vi "GTCP331-200ER - 1.C.(11).vi"(8 "error in (no error)":errorcluster, 11 "RT - Analysis Data in in in":T1={"Accel Sensistivity"=[0.0, 0.0, 0.0], "Cutoff Frequncies"=[{"LP Passband"=0.0, "HP Stopband"=0.0, "LP Stopband"=0.0, "HP Passband"=0.0}, {"LP Passband"=0.0, "HP Stopband"=0.0, "LP Stopband"=0.0, "HP Passband"=0.0}, {"LP Passband"=0.0, "HP Stopband"=0.0, "LP Stopband"=0.0, "HP Passband"=0.0}], "APU Setup File"={"Sensor Info"=[], "Calibration Info"=[], "CMM Table 106"=[], "CMM Table 106B "=[], "Accel Config"=[], "Report Sheet 1"=[], "Report Sheet 2"=[], "Report Sheet 3"=[]}, "RepairLevel"=""} {"Cutoff Frequncies"."HP Passband" min=1.0 step=1.0 format="%#.4f"; "Cutoff Frequncies"."LP Stopband" min=1.0 step=1.0 format="%#.4f"; "Cutoff Frequncies"."HP Stopband" min=1.0 step=1.0 format="%#.4f"; "Cutoff Frequncies"."LP Passband" min=1.0 step=1.0 format="%#.4f"}) -> (0 "error out":errorcluster, 2 "Interactive Mode Vals":dbl[](array[numeric]), 3 "RT - Analysis Data in out":T1 {"Cutoff Frequncies"."HP Passband" min=1.0 step=1.0 format="%#.4f"; "Cutoff Frequncies"."LP Stopband" min=1.0 step=1.0 format="%#.4f"; "Cutoff Frequncies"."HP Stopband" min=1.0 step=1.0 format="%#.4f"; "Cutoff Frequncies"."LP Passband" min=1.0 step=1.0 format="%#.4f"})   [LabVIEW 2018, in "RT - Analysis.lvlib"]
doc: "This subtest perfmors engine run-in procedures."
uses:
  RT - Analysis.lvlib
  Private Controls/Watchdog Settings.ctl
  Private Controls/Interactive Data.ctl
  <vilib>/Analysis/NI_AALBase.lvlib
  <vilib>/Analysis/baseanly.llb/Mean (DBL).vi
  Private Controls/RT-Analysis Data.ctl
  Modules/Testing UI 3/Private Controls/Cutoff Frequency.ctl
  Modules/Testing UI 3/Testing UI 3.lvlib
  Top Level/Shared Controls/APU Setup File.ctl
panel:
  # "Highpass Cutoff Frequency"
  # "Lowpass Cutoff Frequency"
  # "Highpass Cutoff Frequency"
  # "Lowpass Cutoff Frequency"
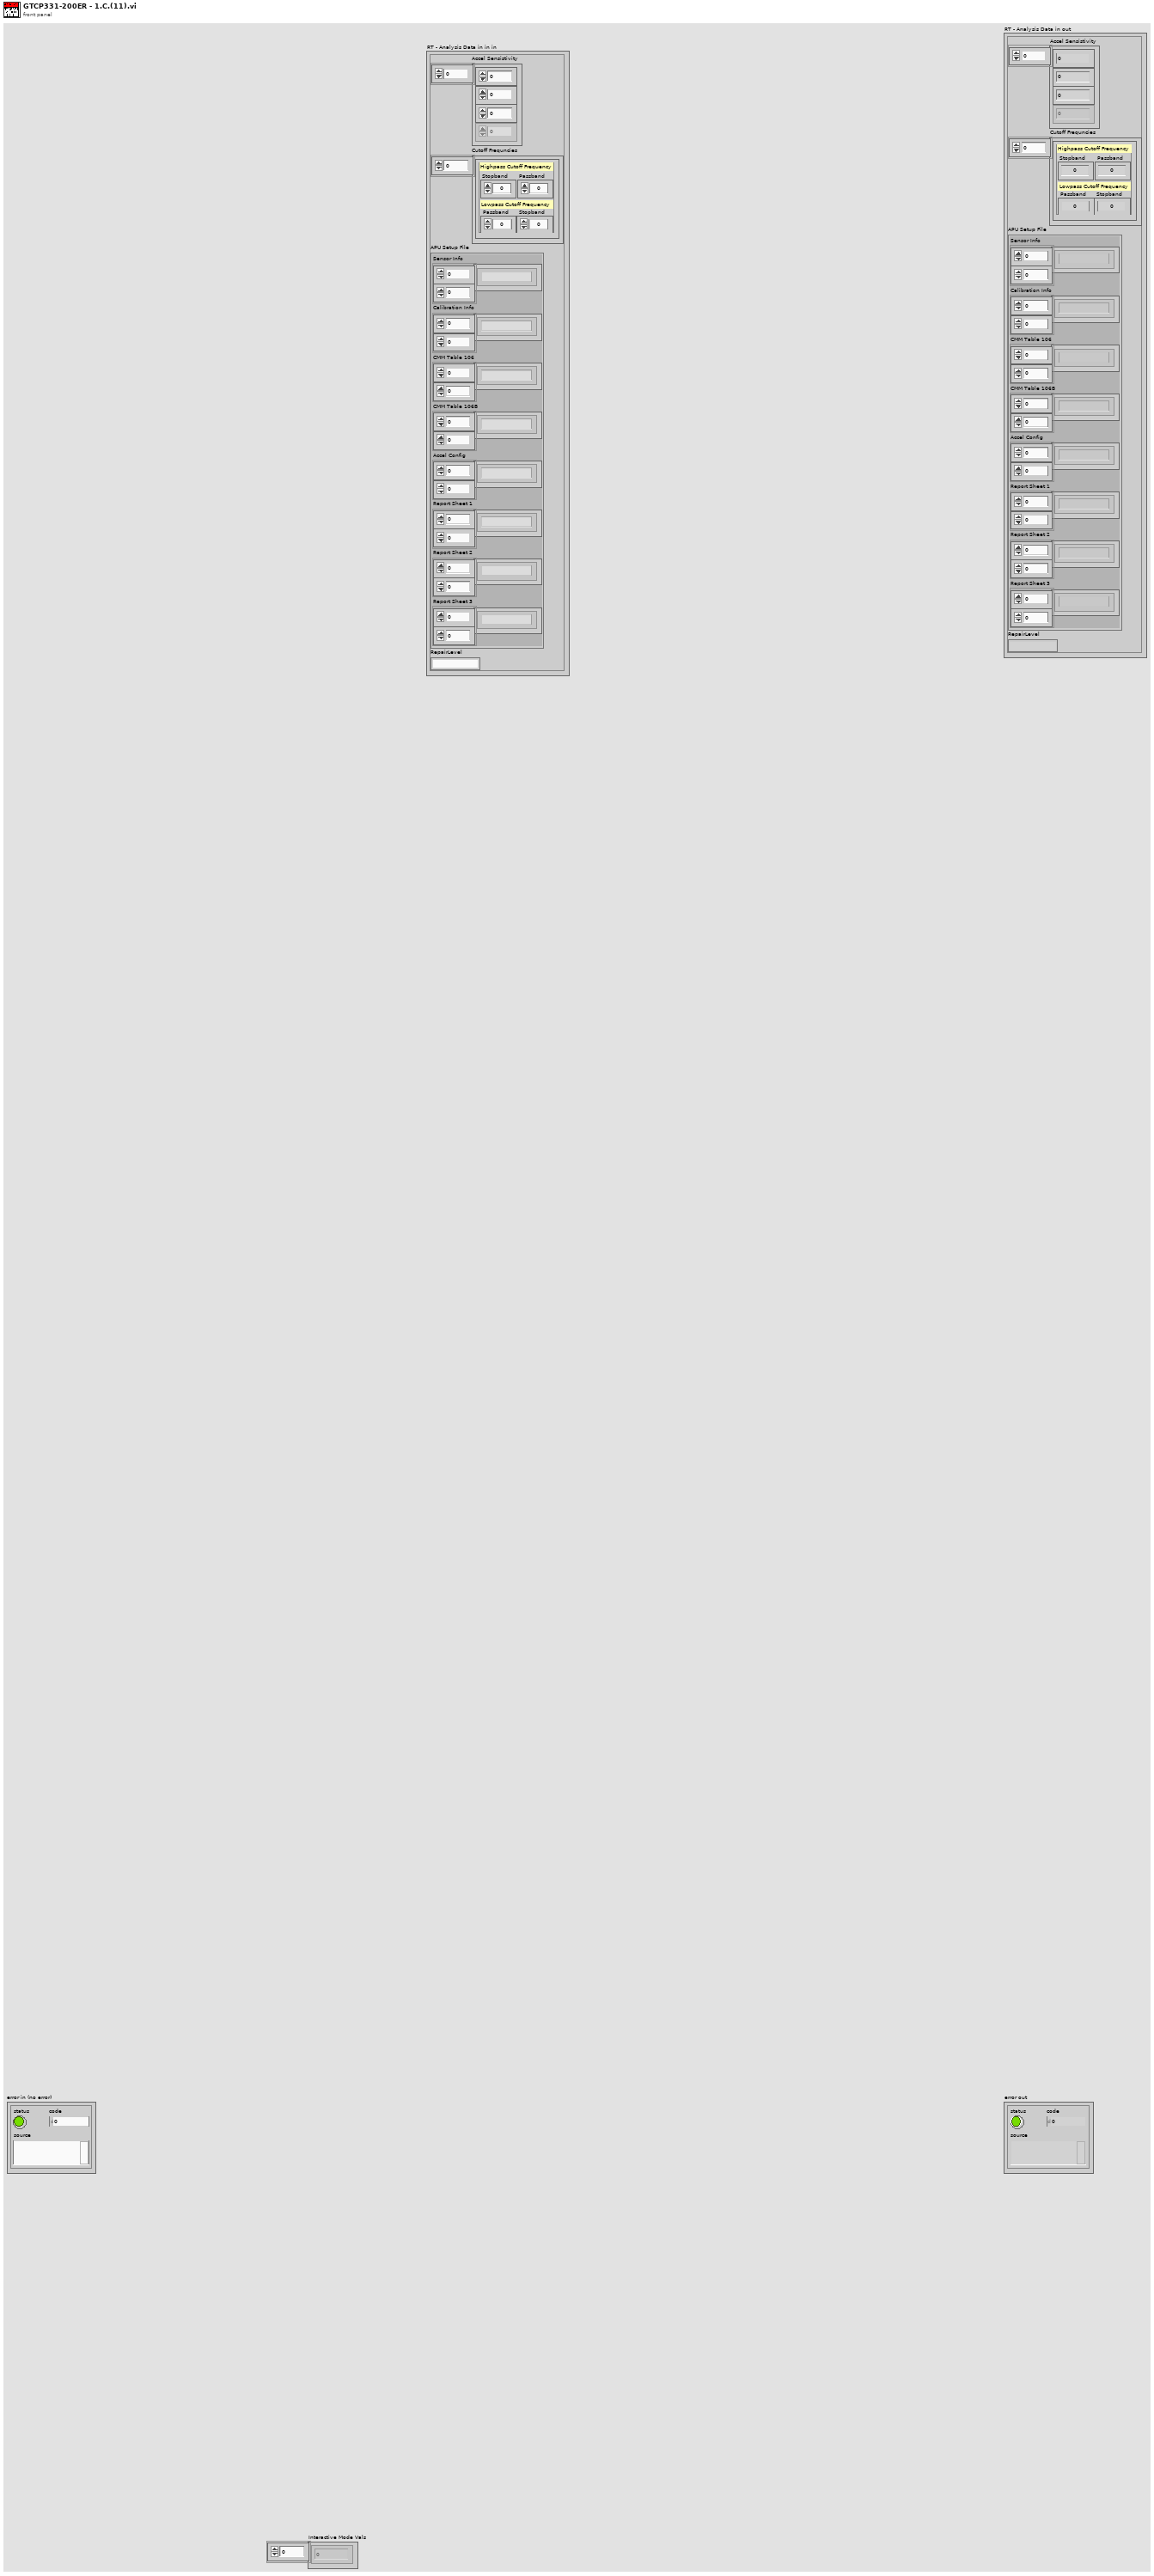
[diagram p1: front panel]
types:
  T1 = typedef "RT - Analysis.lvlib/RT-Analysis Data.ctl" = cluster{"Accel Sensistivity":dbl[], "Cutoff Frequncies":T2[], "APU Setup File":T3, "RepairLevel":string}
  T2 = typedef "Testing UI 3.lvlib/Cutoff Frequency.ctl" = cluster{"LP Passband":dbl, "HP Stopband":dbl, "LP Stopband":dbl, "HP Passband":dbl}
  T3 = typedef "APU Setup File.ctl" = cluster{"Sensor Info":string[][], "Calibration Info":string[][], "CMM Table 106":string[][], "CMM Table 106B ":string[][], "Accel Config":string[][], "Report Sheet 1":string[][], "Report Sheet 2":string[][], "Report Sheet 3":string[][]}
  T4 = typedef "RT - Analysis.lvlib/Watchdog Settings.ctl" = cluster{"Watchdog Action":enum16{"Disabled", "Timer - Change Sample Rate", "RPM Thresh - Insert Other", "RPM Thresh - Check POPD", "RPM Thresh - StartStop Logging"}, "Timer Start":timestamp, "[Watchdog Bools]":bool[], "[Watchdog DBLs]":dbl[], "Watchdog Variant":variant}
  T5 = typedef "RT - Analysis.lvlib/Interactive Data.ctl" = cluster{"Confirm Pressed":bool, "Stored Vals":dbl[]}
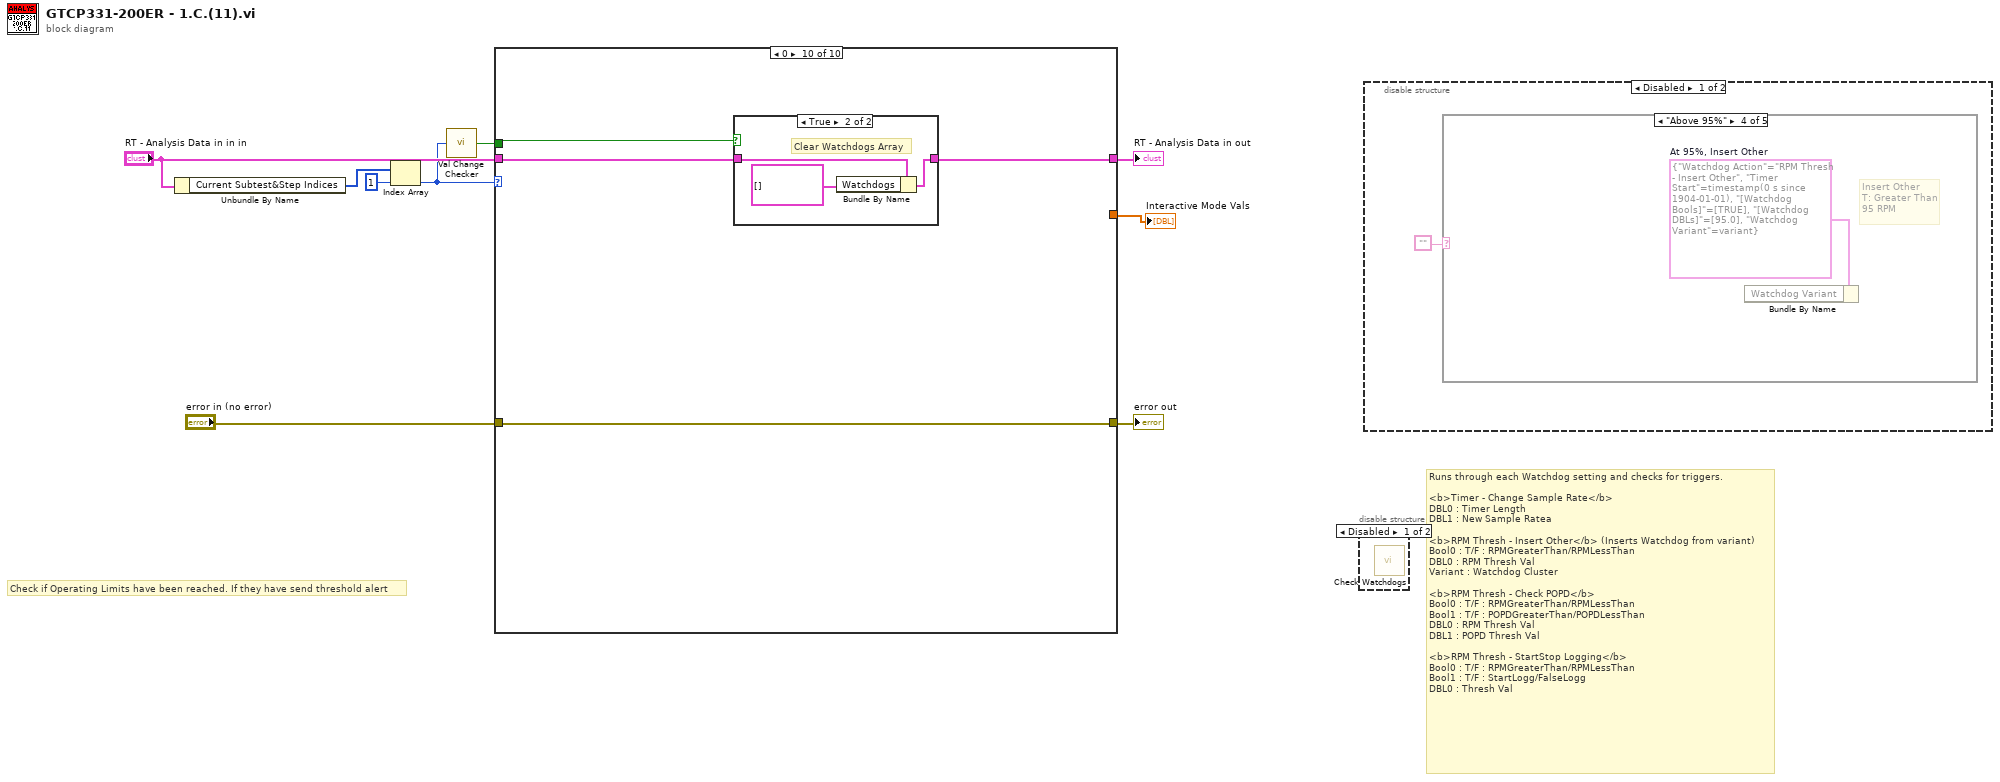
[diagram p0: block diagram]
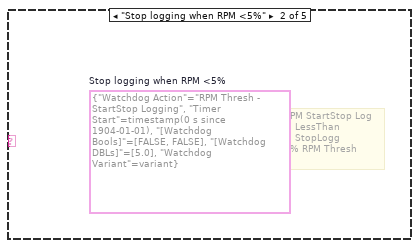
[diagram p3: hidden frame]
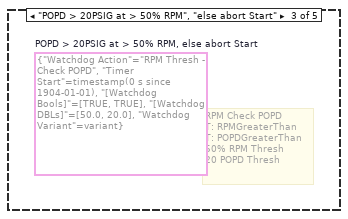
[diagram p4: hidden frame]
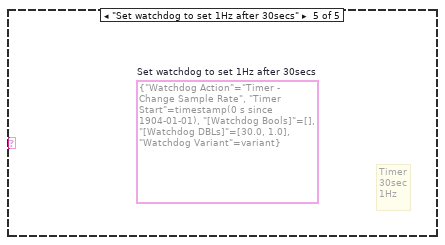
[diagram p5: hidden frame]
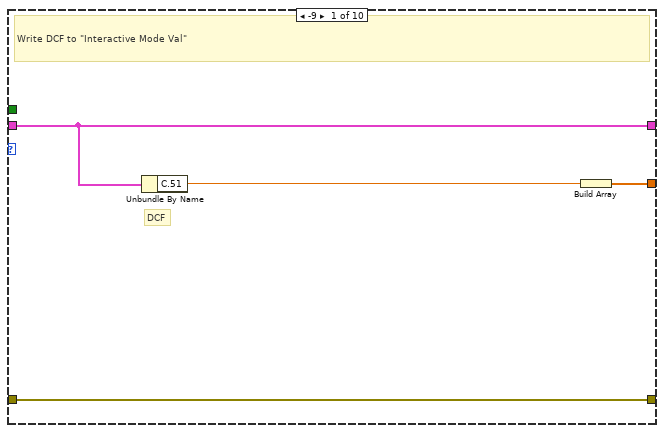
[diagram p8: hidden frame]
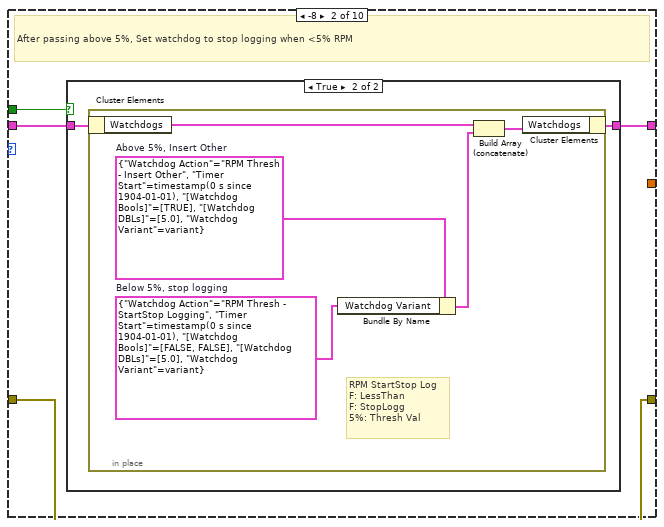
[diagram p9: hidden frame]
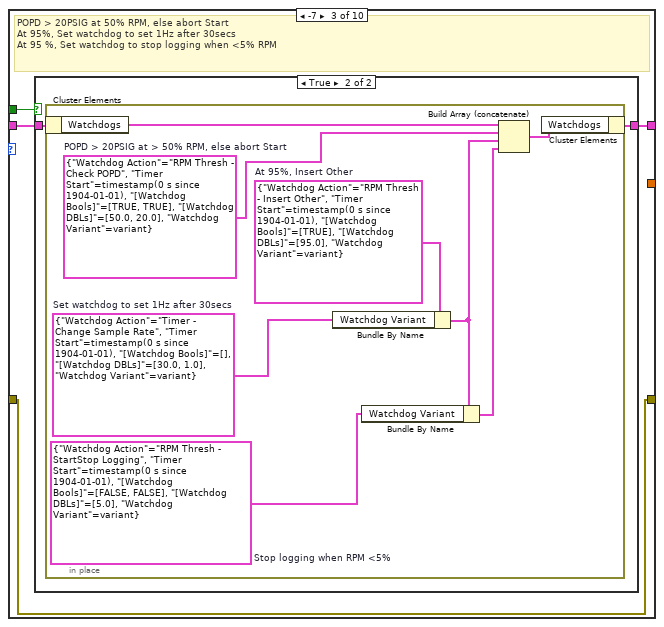
[diagram p11: hidden frame]
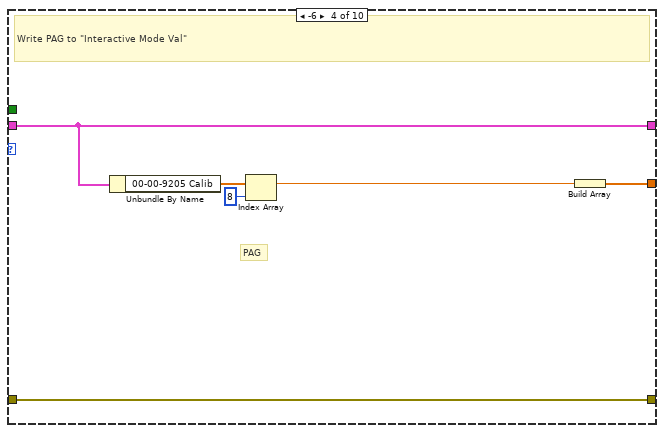
[diagram p13: hidden frame]
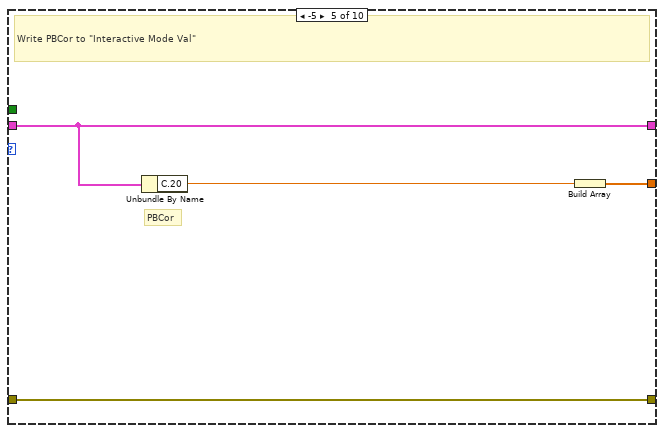
[diagram p14: hidden frame]
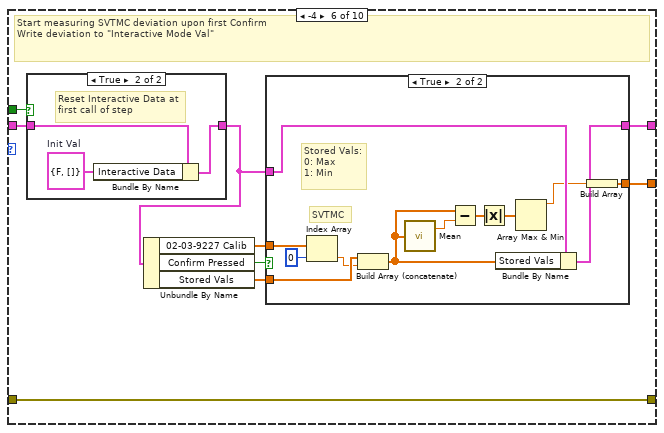
[diagram p15: hidden frame]
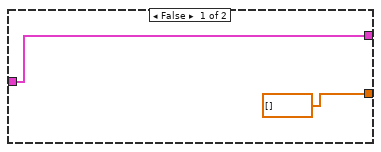
[diagram p16: hidden frame]
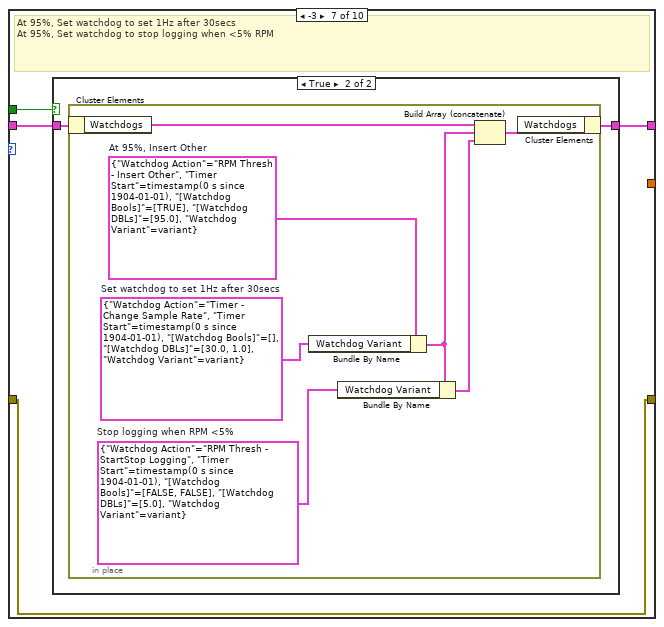
[diagram p18: hidden frame]
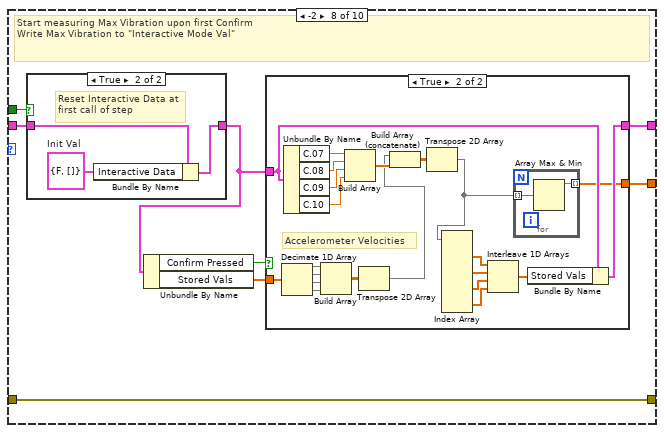
[diagram p20: hidden frame]
diagram:
  # "Runs through each Watchdog setting and checks for triggers.\n\n<b>Timer - Change Sample Rate</b>\nDBL0 : Timer Length\nDBL1 : New Sample Ratea\n\n<b>RPM Thresh - Insert Other</b> (Inserts Watchdog from variant)\nBool0 : T/F : RPMGreaterThan/RPMLessThan\nDBL0 : RPM Thresh Val\nVariant : Watchdog Cluster\n\n<b>RPM Thresh - Check POPD</b>\nBool0 : T/F : RPMGreaterThan/RPMLessThan\nBool1 : T/F : POPDGreaterThan/POPDLessThan\nDBL0 : RPM Thresh Val\nDBL1 : POPD Thresh Val\n\n<b>RPM Thresh - StartStop Logging</b>\nBool0 : T/F : RPMGreaterThan/RPMLessThan\nBool1 : T/F : StartLogg/FalseLogg\nDBL0 : Thresh Val"
  # "Check if Operating Limits have been reached. If they have send threshold alert"
  n1 = Unbundle By Name("RT - Analysis Data in in in") -> ("Current Subtest&Step Indices"=w9:i32[])
  n2 = Index Array(array=w9, index=1) -> (element=w4:i32)
  n3 = call "Val Change Checker.vi"("Current Value in"=w4) -> ("Value Change?"=w3:bool)
  n4 = case shown="0" w4 {
    tunnel: [w13 w17 w29 w46 w50 w59 w81 w99 w132 w136] -> w7
    tunnel: "error in (no error)" -> [w13 w17 w29 w46 w50 w59 w81 w99 w132 w136]
    tunnel: [w12 w16 w28 w45 w49 w52 w80 w92 w131 w133] -> w6
    tunnel: "RT - Analysis Data in in in" -> [w12 w15 w27 w45 w49 w56 w79 w96 w131 w134]
    tunnel: [w10 _ _ w43 w47 w58 _ w98 dbl[] [] ("Interactive Mode Vals") _] -> w1
    tunnel: w3 -> [_ w14 w26 _ _ w57 w78 w97 _ w135]
    frame -9 {
      # "DCF"
      # "Write DCF to \"Interactive Mode Val\""
      n5 = Unbundle By Name(w12) -> ("C.51"=w11:dbl)
      n6 = Build Array(w11) -> (w10:dbl[])
    }
    frame -8 {
      # "After passing above 5%, Set watchdog to stop logging when <5% RPM"
      n7 = case shown="True" w14 {
        tunnel: [w18 w20] -> w16
        tunnel: w15 -> [w18 w19]
        frame False {
        }
        frame True {
          n8 = in-place {
            w21 = T4 {"Watchdog Action"=enum."RPM Thresh - StartStop Logging", "Timer Start"=timestamp(0 s since 1904-01-01), "[Watchdog Bools]"=[FALSE, FALSE], "[Watchdog DBLs]"=[5.0], "Watchdog Variant"=variant}  # Below 5%, stop logging
            w23 = T4 {"Watchdog Action"=enum."RPM Thresh - Insert Other", "Timer Start"=timestamp(0 s since 1904-01-01), "[Watchdog Bools]"=[TRUE], "[Watchdog DBLs]"=[5.0], "Watchdog Variant"=variant}  # Above 5%, Insert Other
            # "RPM StartStop Log\nF: LessThan\nF: StopLogg\n5%: Thresh Val"
            n9 = in-place-cluster #1(w19) -> ("Watchdogs"=w24:T4[])
            n10 = Bundle By Name(cluster=w23, "Watchdog Variant"=w21) -> (w22:T4)
            n11 = Build Array (concatenate)(w24, w22) -> (w25:T4[])
            n12 = in-place-cluster #1("Watchdogs"=w25) -> (w20:T1)
          }
        }
      }
    }
    frame -7 {
      # "POPD > 20PSIG at 50% RPM, else abort Start\nAt 95%, Set watchdog to set 1Hz after 30secs\nAt 95 %, Set watchdog to stop logging when <5% RPM"
      n13 = case shown="True" w26 {
        tunnel: [w30 w32] -> w28
        tunnel: w27 -> [w30 w31]
        frame False {
        }
        frame True {
          n14 = in-place {
            w33 = T4 {"Watchdog Action"=enum."RPM Thresh - StartStop Logging", "Timer Start"=timestamp(0 s since 1904-01-01), "[Watchdog Bools]"=[FALSE, FALSE], "[Watchdog DBLs]"=[5.0], "Watchdog Variant"=variant}  # Stop logging when RPM <5%
            w38 = T4 {"Watchdog Action"=enum."Timer - Change Sample Rate", "Timer Start"=timestamp(0 s since 1904-01-01), "[Watchdog Bools]"=[], "[Watchdog DBLs]"=[30.0, 1.0], "Watchdog Variant"=variant}  # Set watchdog to set 1Hz after 30secs
            w37 = T4 {"Watchdog Action"=enum."RPM Thresh - Insert Other", "Timer Start"=timestamp(0 s since 1904-01-01), "[Watchdog Bools]"=[TRUE], "[Watchdog DBLs]"=[95.0], "Watchdog Variant"=variant}  # At 95%, Insert Other
            w36 = T4 {"Watchdog Action"=enum."RPM Thresh - Check POPD", "Timer Start"=timestamp(0 s since 1904-01-01), "[Watchdog Bools]"=[TRUE, TRUE], "[Watchdog DBLs]"=[50.0, 20.0], "Watchdog Variant"=variant}  # POPD > 20PSIG at > 50% RPM, else abort Start
            n15 = in-place-cluster #2(w31) -> ("Watchdogs"=w39:T4[])
            n16 = Bundle By Name(cluster=w37, "Watchdog Variant"=w38) -> (w35:T4)
            n17 = Bundle By Name(cluster=w35, "Watchdog Variant"=w33) -> (w34:T4)
            n18 = Build Array (concatenate)(w39, w36, w35, w34) -> (w40:T4[])
            n19 = in-place-cluster #2("Watchdogs"=w40) -> (w32:T1)
          }
        }
      }
    }
    frame -6 {
      # "PAG"
      # "Write PAG to \"Interactive Mode Val\""
      n20 = Unbundle By Name(w45) -> ("00-00-9205 Calib"=w44:dbl[])
      n21 = Index Array(array=w44, index=8) -> (element=w42:dbl)
      n22 = Build Array(w42) -> (w43:dbl[])
    }
    frame -5 {
      # "PBCor"
      # "Write PBCor to \"Interactive Mode Val\""
      n23 = Unbundle By Name(w49) -> ("C.20"=w48:dbl)
      n24 = Build Array(w48) -> (w47:dbl[])
    }
    frame -4 {
      # "Start measuring SVTMC deviation upon first Confirm\nWrite deviation to \"Interactive Mode Val\""
      n25 = case shown="True" w57 {
        tunnel: w56 -> [w74 w77]
        tunnel: [w74 w76] -> w55
        frame False {
        }
        frame True {
          w75 = T5 {"Confirm Pressed"=FALSE, "Stored Vals"=[]}  # Init Val
          # "Reset Interactive Data at\nfirst call of step"
          n26 = Bundle By Name(cluster=w77, "Interactive Data"=w75) -> (w76:T1)
        }
      }
      n27 = Unbundle By Name(w55) -> ("02-03-9227 Calib"=w51:dbl[], "Confirm Pressed"=w54:bool, "Stored Vals"=w53:dbl[])
      n28 = case shown="True" w54 {
        tunnel: [dbl[] [] ("Interactive Mode Vals") w62] -> w58
        tunnel: w55 -> [w61 w73]
        tunnel: w53 -> [_ w69]
        tunnel: [w61 w72] -> w52
        tunnel: w51 -> [_ w71]
        frame False {
        }
        frame True {
          # "Stored Vals:\n0: Max\n1: Min"
          # "SVTMC"
          n29 = Index Array(array=w71, index=0) -> (element=w68:dbl)
          n30 = Build Array (concatenate)(w69, w68) -> (w66:dbl[])
          n31 = call-poly <vilib>:"Mean.vi"("X"=w66) -> ("mean"=w67:dbl)  [unwired: 1 out]
          n32 = Subtract(x=w66, y=w67) -> (x-y=w65:dbl[])
          n33 = Absolute Value(x=w65) -> (abs(x)=w64:dbl[])
          n34 = Bundle By Name(cluster=w73, "Stored Vals"=w66) -> (w72:T1)
          n35 = Array Max & Min(array=w64) -> (max value=w63:dbl)  [unwired: 3 out]
          n36 = Build Array(w63) -> (w62:dbl[])
        }
      }
    }
    frame -3 {
      # "At 95%, Set watchdog to set 1Hz after 30secs\nAt 95%, Set watchdog to stop logging when <5% RPM"
      n37 = case shown="True" w78 {
        tunnel: [w82 w84] -> w80
        tunnel: w79 -> [w82 w83]
        frame False {
        }
        frame True {
          n38 = in-place {
            w85 = T4 {"Watchdog Action"=enum."RPM Thresh - StartStop Logging", "Timer Start"=timestamp(0 s since 1904-01-01), "[Watchdog Bools]"=[FALSE, FALSE], "[Watchdog DBLs]"=[5.0], "Watchdog Variant"=variant}  # Stop logging when RPM <5%
            w89 = T4 {"Watchdog Action"=enum."Timer - Change Sample Rate", "Timer Start"=timestamp(0 s since 1904-01-01), "[Watchdog Bools]"=[], "[Watchdog DBLs]"=[30.0, 1.0], "Watchdog Variant"=variant}  # Set watchdog to set 1Hz after 30secs
            w88 = T4 {"Watchdog Action"=enum."RPM Thresh - Insert Other", "Timer Start"=timestamp(0 s since 1904-01-01), "[Watchdog Bools]"=[TRUE], "[Watchdog DBLs]"=[95.0], "Watchdog Variant"=variant}  # At 95%, Insert Other
            n39 = in-place-cluster #3(w83) -> ("Watchdogs"=w90:T4[])
            n40 = Bundle By Name(cluster=w88, "Watchdog Variant"=w89) -> (w87:T4)
            n41 = Bundle By Name(cluster=w87, "Watchdog Variant"=w85) -> (w86:T4)
            n42 = Build Array (concatenate)(w90, w87, w86) -> (w91:T4[])
            n43 = in-place-cluster #3("Watchdogs"=w91) -> (w84:T1)
          }
        }
      }
    }
    frame -2 {
      # "Start measuring Max Vibration upon first Confirm\nWrite Max Vibration to \"Interactive Mode Val\""
      n44 = case shown="True" w97 {
        tunnel: w96 -> [w126 w129]
        tunnel: [w126 w128] -> w95
        frame False {
        }
        frame True {
          w127 = T5 {"Confirm Pressed"=FALSE, "Stored Vals"=[]}  # Init Val
          # "Reset Interactive Data at\nfirst call of step"
          n45 = Bundle By Name(cluster=w129, "Interactive Data"=w127) -> (w128:T1)
        }
      }
      n46 = Unbundle By Name(w95) -> ("Confirm Pressed"=w94:bool, "Stored Vals"=w93:dbl[])
      n47 = case shown="True" w94 {
        tunnel: [dbl[] [] ("Interactive Mode Vals") w107] -> w98
        tunnel: w95 -> [w101 w117]
        tunnel: w93 -> [_ w122]
        tunnel: [w101 w123] -> w92
        frame False {
        }
        frame True {
          # "Accelerometer Velocities"
          n48 = Decimate 1D Array(w122) -> (w121:dbl[], w120:dbl[], w119:dbl[], w116:dbl[])
          n49 = Unbundle By Name(w117) -> ("C.07"=w111:dbl, "C.08"=w110:dbl, "C.09"=w109:dbl, "C.10"=w108:dbl)
          n50 = Build Array(w121, w120, w119, w116) -> (w105:dbl[][])
          n51 = Build Array(w111, w110, w109, w108) -> (w106:dbl[])
          n52 = Transpose 2D Array(2D array=w105) -> (transposed array=w102:dbl[][])
          n53 = Build Array (concatenate)(w102, w106) -> (w104:dbl[][])
          n54 = Transpose 2D Array(2D array=w104) -> (transposed array=w103:dbl[][])
          n55 = Index Array(array=w103) -> (element #1=w115:dbl[], element #2=w114:dbl[], element #3=w113:dbl[], element #4=w112:dbl[])  [unwired: 8 in]
          n56 = Interleave 1D Arrays(w115, w114, w113, w112) -> (w118:dbl[])
          n57 = for {
            tunnel: [w125] -> w107 mode=indexing
            tunnel: w103 -> [w124] mode=indexing
            n58 = Array Max & Min(array=w124) -> (max value=w125:dbl)  [unwired: 3 out]
          }
          n59 = Bundle By Name(cluster=w117, "Stored Vals"=w118) -> (w123:T1)
        }
      }
    }
    frame -1, Default {
      # "Unused Index"
    }
    frame 0 {
      n60 = case shown="True" w135 {
        tunnel: w134 -> [w137 w140]
        tunnel: [w137 w139] -> w133
        frame False {
        }
        frame True {
          # "Clear Watchdogs Array"
          n61 = Bundle By Name(cluster=w140, "Watchdogs"=T4[] []) -> (w139:T1)
        }
      }
    }
  }
  "RT - Analysis Data in out" <- w6
  "error out" <- w7
  "Interactive Mode Vals" <- w1
  n62 = disable-structure shown="Disabled" {
    frame Disabled {
      n63 = call "Check Watchdogs.vi"() -> ()  [unwired: 10 in, 2 out]
    }
    frame Enabled {
    }
  }
  n64 = disable-structure shown="Disabled" {
    frame Disabled {
      n65 = case shown="\"Above 95%\"" "" {
        frame Default {
        }
        frame "Stop logging when RPM <5%" {
          (unwired) T4 {"Watchdog Action"=enum."RPM Thresh - StartStop Logging", "Timer Start"=timestamp(0 s since 1904-01-01), "[Watchdog Bools]"=[FALSE, FALSE], "[Watchdog DBLs]"=[5.0], "Watchdog Variant"=variant}  # Stop logging when RPM <5%
          # "RPM StartStop Log\nF: LessThan\nF: StopLogg\n5% RPM Thresh"
        }
        frame "POPD > 20PSIG at > 50% RPM", "else abort Start" {
          (unwired) T4 {"Watchdog Action"=enum."RPM Thresh - Check POPD", "Timer Start"=timestamp(0 s since 1904-01-01), "[Watchdog Bools]"=[TRUE, TRUE], "[Watchdog DBLs]"=[50.0, 20.0], "Watchdog Variant"=variant}  # POPD > 20PSIG at > 50% RPM, else abort Start
          # "RPM Check POPD\nT: RPMGreaterThan\nT: POPDGreaterThan\n50% RPM Thresh\n20 POPD Thresh"
        }
        frame "Above 95%" {
          w142 = T4 {"Watchdog Action"=enum."RPM Thresh - Insert Other", "Timer Start"=timestamp(0 s since 1904-01-01), "[Watchdog Bools]"=[TRUE], "[Watchdog DBLs]"=[95.0], "Watchdog Variant"=variant}  # At 95%, Insert Other
          # "Insert Other\nT: Greater Than\n95 RPM"
          n66 = Bundle By Name(cluster=w142) -> ()  [unwired: 1 in, 1 out]
        }
        frame "Set watchdog to set 1Hz after 30secs" {
          (unwired) T4 {"Watchdog Action"=enum."Timer - Change Sample Rate", "Timer Start"=timestamp(0 s since 1904-01-01), "[Watchdog Bools]"=[], "[Watchdog DBLs]"=[30.0, 1.0], "Watchdog Variant"=variant}  # Set watchdog to set 1Hz after 30secs
          # "Timer\n30sec\n1Hz"
        }
      }
    }
    frame Enabled {
    }
  }
